vi "Motion Profile Generator-Demo.vi"(0 "Max Speed (rotations/sec)":dbl=3.0, 5 "Max Acceleration (rotations/sec^2)":dbl=1.0, 7 "Max Jerk (rotations/sec^3)":dbl=1.0, 9 "Rotations to Travel":dbl=4.0, 11 "Motion Profile Control Frame Rate":dbl=10.0) -> (4 "Position rotations":dbl[](array[numeric]), 6 "velocity rotations/sec":dbl[](array[numeric]), 8 "acceleration rotations/sec^2":dbl[](array[numeric]), 10 "XY Graph":cluster{dbl[], dbl[]}[](graph))   [LabVIEW 2015]
panel:
  out "Final Position":dbl
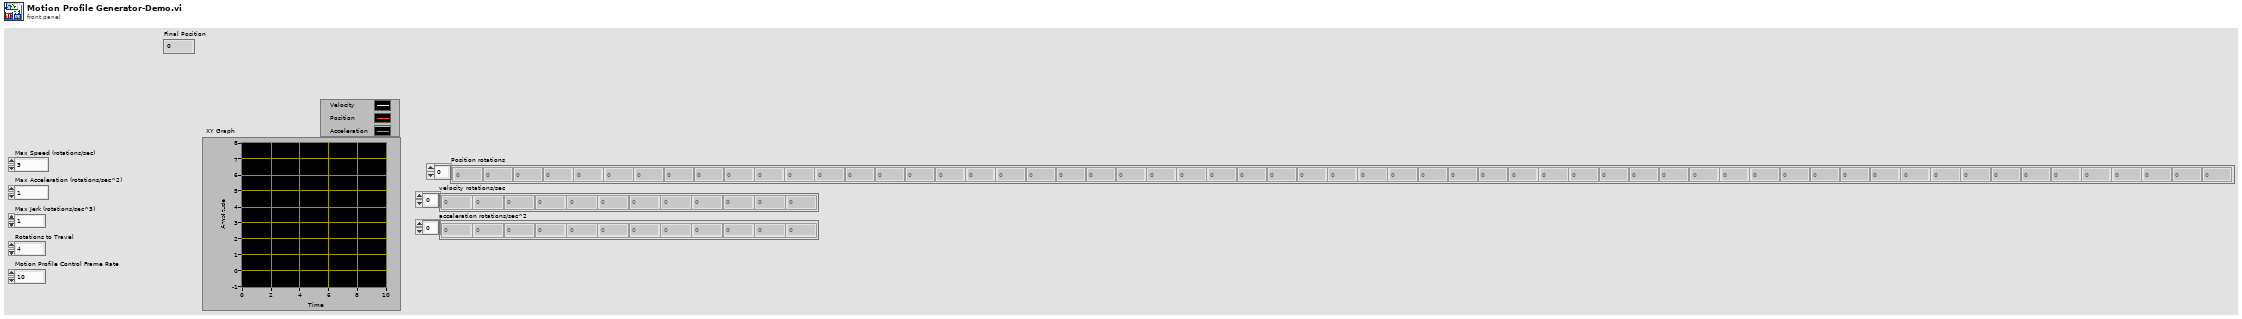
[diagram p1: front panel]
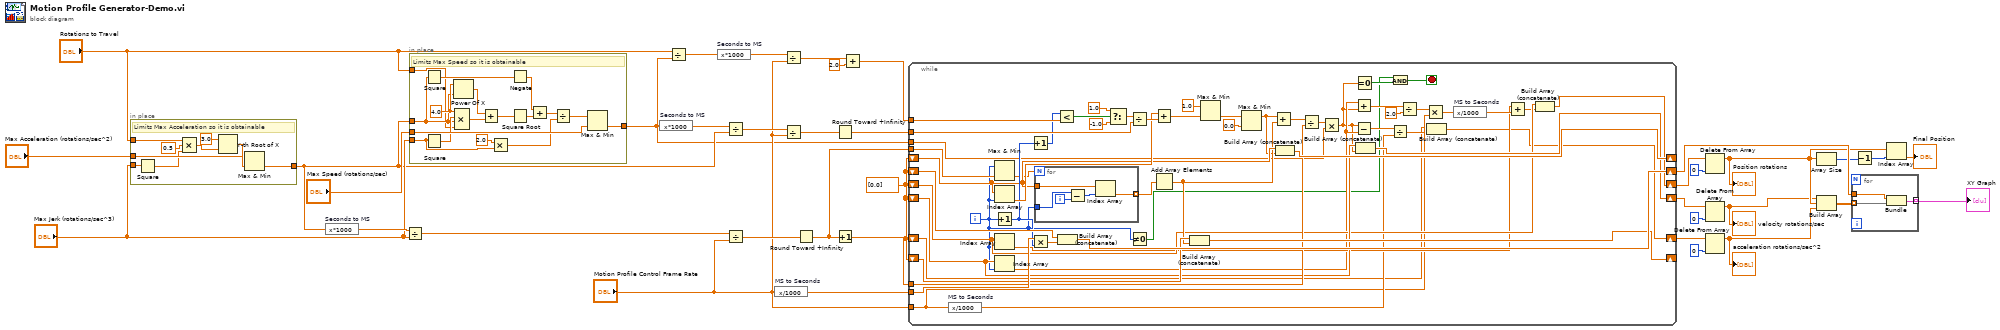
[diagram p0: block diagram]
diagram:
  w22 = dbl[] [0.0]
  n1 = in-place {
    in-place-border: "Max Jerk (rotations/sec^3)" -> [w47]
    in-place-border: "Max Acceleration (rotations/sec^2)" -> [w45]
    in-place-border: [w44] -> w12
    in-place-border: "Rotations to Travel" -> [w43]
    # "Limits Max Acceleration so it is obtainable"
    n2 = Square(x=w47) -> (x^2=w41:dbl)
    n3 = Compound Arithmetic op=MULTIPLY(w43, 0.5 ("value"), w41) -> (w40:dbl)
    n4 = Y-th Root of X(1:w40, 2:3.0 ("y")) -> (0:w46:dbl)
    n5 = Max & Min(x=w45, y=w46) -> (min(x,y)=w44:dbl)  [unwired: 1 out]
  }
  n6 = expression code="x*1000" "Seconds to MS"(w12) -> (w37:dbl)
  n7 = Divide(x=w37, y="Max Jerk (rotations/sec^3)") -> (x/y=w27:dbl)
  n8 = in-place {
    in-place-border: "Max Speed (rotations/sec)" -> [w64]
    in-place-border: [w51] -> w11
    in-place-border: w12 -> [w57]
    in-place-border: "Rotations to Travel" -> [w56]
    in-place-border: "Max Jerk (rotations/sec^3)" -> [w53]
    w60 = 4.0 ("x")
    # "Limits Max Speed so it is obtainable"
    n9 = Square(x=w57) -> (x^2=w63:dbl)
    n10 = Square(x=w53) -> (x^2=w59:dbl)
    n11 = Power Of X(1:w57, 2:w60) -> (0:w61:dbl)
    n12 = Compound Arithmetic op=MULTIPLY(w60, w59, w57, w56) -> (w58:dbl)
    n13 = Add(x=w61, y=w58) -> (x+y=w55:dbl)
    n14 = Multiply(x=2.0, y=w53) -> (x*y=w48:dbl)
    n15 = Negate(x=w63) -> (-x=w62:dbl)
    n16 = Square Root(x=w55) -> (sqrt(x)=w52:dbl)
    n17 = Add(x=w62, y=w52) -> (x+y=w50:dbl)
    n18 = Divide(x=w50, y=w48) -> (x/y=w49:dbl)
    n19 = Max & Min(x=w49, y=w64) -> (min(x,y)=w51:dbl)  [unwired: 1 out]
  }
  n20 = expression code="x*1000" "Seconds to MS"(w11) -> (w36:dbl)
  n21 = Divide(x="Rotations to Travel", y=w11) -> (x/y=w35:dbl)
  n22 = expression code="x*1000" "Seconds to MS"(w35) -> (w34:dbl)
  n23 = Divide(x=w36, y=w12) -> (x/y=w30:dbl)
  n24 = Divide(x=w27, y="Motion Profile Control Frame Rate") -> (x/y=w26:dbl)
  n25 = expression code="x/1000" "MS to Seconds"("Motion Profile Control Frame Rate") -> (w38:dbl)
  n26 = Divide(x=w34, y="Motion Profile Control Frame Rate") -> (x/y=w33:dbl)
  n27 = Divide(x=w30, y="Motion Profile Control Frame Rate") -> (x/y=w29:dbl)
  n28 = Round Toward +Infinity(x=w26) -> (ceil(x): smallest int >= x=w25:dbl)
  n29 = Round Toward +Infinity(x=w29) -> (ceil(x): smallest int >= x=w28:dbl)
  n30 = Increment(x=w25) -> (x+1=w24:dbl)
  n31 = Add(x=w33, y=2.0) -> (x+y=w31:dbl)
  n32 = while {
    shift-right: [w117] -> w20
    shift-left: w22 -> [w118]
    tunnel: w38 -> [w116]
    tunnel: w31 -> [w114]
    shift-right: [w100] -> _
    shift-left: w22 -> [w99]
    tunnel: w28 -> [w106]
    tunnel: w25 -> [w97]
    shift-right: [w94] -> _
    shift-left: w22 -> [w95]
    tunnel: w24 -> [w90]
    tunnel: w11 -> [w88]
    shift-right: [w87] -> w5
    shift-left: w22 -> [w85]
    shift-right: [w86] -> w3
    shift-left: w22 -> [w79]
    tunnel: "Motion Profile Control Frame Rate" -> [w73]
    shift-right: [w71] -> w7
    shift-left: w22 -> [w70]
    i -> [w69]
    stop <- w65 stop-if-true
    n33 = expression code="x/1000" "MS to Seconds"(w73) -> (w74:dbl)
    n34 = Max & Min(x=w69, y=w97) -> (min(x,y)=w96:dbl)  [unwired: 1 out]
    n35 = Index Array(array=w99, index=w69) -> (element=w104:dbl)
    n36 = Increment(x=w69) -> (x+1=w102:i32)
    n37 = Index Array(array=w79, index=w69) -> (element=w78:dbl)
    n38 = Index Array(array=w85, index=w69) -> (element=w76:dbl)
    n39 = Increment(x=w102) -> (x+1=w103:i32)
    n40 = Multiply(x=w116, y=w102) -> (x*y=w115:dbl)
    n41 = for {
      N: w96 -> [_]
      tunnel: w69 -> [w122]
      tunnel: w99 -> [w120]
      tunnel: [w119] -> w98 mode=indexing
      i -> [w123]
      n42 = Subtract(x=w122, y=w123) -> (x-y=w121:i32)
      n43 = Index Array(array=w120, index=w121) -> (element=w119:dbl)
    }
    n44 = Less?(x=w103, y=w114) -> (x < y?=w110:bool)
    n45 = Build Array (concatenate)(w118, w115) -> (w117:dbl[])
    n46 = Select(t=1.0, s=w110, f=-1.0) -> (s? t:f=w107:dbl)
    n47 = Divide(x=w107, y=w106) -> (x/y=w105:dbl)
    n48 = Not Equal To 0?(x=w69) -> (x != 0?=w66:bool)
    n49 = Add(x=w104, y=w105) -> (x+y=w101:dbl)
    n50 = Add Array Elements(numeric array=w98) -> (sum=w93:dbl)
    n51 = Build Array (concatenate)(w95, w93) -> (w94:dbl[])
    n52 = Max & Min(x=1.0, y=w101) -> (min(x,y)=w112:dbl)  [unwired: 1 out]
    n53 = Max & Min(x=w112, y=0.0) -> (max(x,y)=w92:dbl)  [unwired: 1 out]
    n54 = Add(x=w92, y=w93) -> (x+y=w91:dbl)
    n55 = Build Array (concatenate)(w99, w92) -> (w100:dbl[])
    n56 = Divide(x=w91, y=w90) -> (x/y=w89:dbl)
    n57 = Multiply(x=w89, y=w88) -> (x*y=w68:dbl)
    n58 = Add(x=w76, y=w68) -> (x+y=w84:dbl)
    n59 = Subtract(x=w68, y=w76) -> (x-y=w75:dbl)
    n60 = Equal To 0?(x=w68) -> (x = 0?=w67:bool)
    n61 = Build Array (concatenate)(w85, w68) -> (w87:dbl[])
    n62 = Divide(x=w75, y=w74) -> (x/y=w72:dbl)
    n63 = And(x=w66, y=w67) -> (x .and. y?=w65:bool)
    n64 = Divide(x=w84, y=2.0) -> (x/y=w82:dbl)
    n65 = Multiply(x=w82, y=w73) -> (x*y=w81:dbl)
    n66 = Build Array (concatenate)(w70, w72) -> (w71:dbl[])
    n67 = expression code="x/1000" "MS to Seconds"(w81) -> (w80:dbl)
    n68 = Add(x=w78, y=w80) -> (x+y=w77:dbl)
    n69 = Build Array (concatenate)(w79, w77) -> (w86:dbl[])
  }
  n70 = Delete From Array(array=w3, index=0) -> (array with subset deleted=w2:dbl[])  [unwired: 1 in, 1 out]
  "Position rotations" <- w2
  n71 = Delete From Array(array=w5, index=0) -> (array with subset deleted=w1:dbl[])  [unwired: 1 in, 1 out]
  "velocity rotations/sec" <- w1
  n72 = Delete From Array(array=w7, index=0) -> (array with subset deleted=w6:dbl[])  [unwired: 1 in, 1 out]
  "acceleration rotations/sec^2" <- w6
  n73 = Array Size(array=w2) -> (size(s)=w18:i32)
  n74 = Build Array(w1, w2, w6) -> (w21:dbl[][])
  n75 = for {
    tunnel: w21 -> [w126] mode=indexing
    tunnel: w20 -> [w125]
    tunnel: [w124] -> w19 mode=indexing
    n76 = Bundle(w125, w126) -> (w124:cluster{dbl[], dbl[]})  [unwired: 1 in]
  }
  "XY Graph" <- w19
  n77 = Decrement(x=w18) -> (x-1=w17:i32)
  n78 = Index Array(array=w2, index=w17) -> (element=→"Final Position":dbl)
